vi "Send Dialog Return Msg.vi"(8 "error in (no error)":errorcluster, 11 "Dialog Return Msg":refnum<class "Dialog Return Msg.lvclass">) -> (0 "error out":errorcluster)   [LabVIEW 2017, in "IDialogBox.lvlib" / "Dialog Return Msg.lvclass"]
uses:
  <vilib>/gpm_packages/@cs/mva-dialogbox/source/IDialogBox/IDialogBox Messages/Dialog Return Msg/Dialog Return Msg.lvclass
  C:/Program Files/National Instruments/LabVIEW 2017/vi.lib/gpm_packages/@cs/actor-framework-messages/Source/RoundTripMessage/RoundTripMessage.lvclass
  <vilib>/gpm_packages/@cs/actor-framework-messages/Source/RoundTripMessage/RoundTripMessage.lvclass/RoundTripMessage.ctl
  <vilib>/ActorFramework/Message Enqueuer/Message Enqueuer.lvclass/Message Enqueuer.ctl
  <vilib>/ActorFramework/Message Enqueuer/Enqueue.vi
  <vilib>/gpm_packages/@cs/actor-framework-messages/Source/RoundTripMessage/RoundTripMessage.lvclass
  C:/Program Files/National Instruments/LabVIEW 2017/vi.lib/ActorFramework/Message/Message.lvclass
  <vilib>/ActorFramework/Message Priority Queue/Priority Enqueue.vi
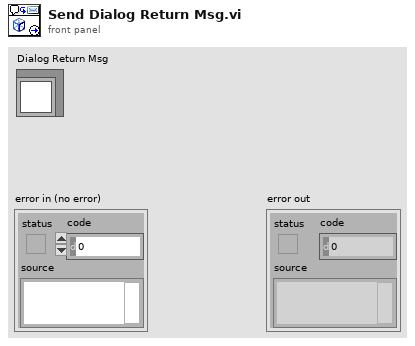
[diagram p1: front panel]
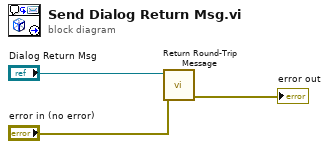
[diagram p0: block diagram]
diagram:
  n1 = call <vilib>:"Return Round-Trip Message.vi"("error in (no error)"="error in (no error)", "RoundTripMessage In"="Dialog Return Msg") -> ("error out"=→"error out":errorcluster)  [unwired: 9 in]
